vi "RedP--reader--V1.vi"() -> ()   [LabVIEW 2018]
uses:
  MFLI frontend action.ctl
  mfli reader event.ctl
  RedPitaSettings.ctl
  NHMFL_Core/Libraries/Red Pitaya/RP Core/RP Transceiver/RP Transceiver.lvclass
  publisher action.ctl
panel:
  in  "stop  !":bool
  in  "start  !":bool
  in  "all":enum32{"all"}(tab)
  out "read Voltage (V)":cdb=3.4008953474285613e-07-2.099650132525618e-08i format="%#10_10f"
  in  "read status":bool
  out "read Voltage X (V)":dbl=3.4008953474285613e-07 format="%#11_11f"
  out "read Voltage Y (V)":dbl=-2.099650132525618e-08 format="%#11_11f"
  in  "delay-read (msec)":u32=200
  out "zi freq (Hz)":dbl=59582.54261216211 format="%-#.3f"
  in  "red pita ip  Address":string="146.201.232.88"
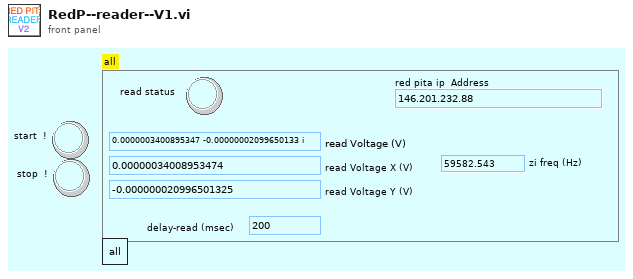
[diagram p1: front panel]
types:
  T1 = typedef "RedPitaSettings.ctl" = cluster{"time constant":dbl, "RP Transeiver":refnum<class "RP Transceiver.lvclass">, "samples per read":i32, "IP address":string}
  T2 = typedef "MFLI frontend action.ctl" = enum16{"read", "writeread", "open", "close", "write"}
  T3 = typedef "mfli reader event.ctl" = enum16{"start", "stop"}
  T4 = typedef "publisher action.ctl" = enum16{"set", "get", "init", "check"}
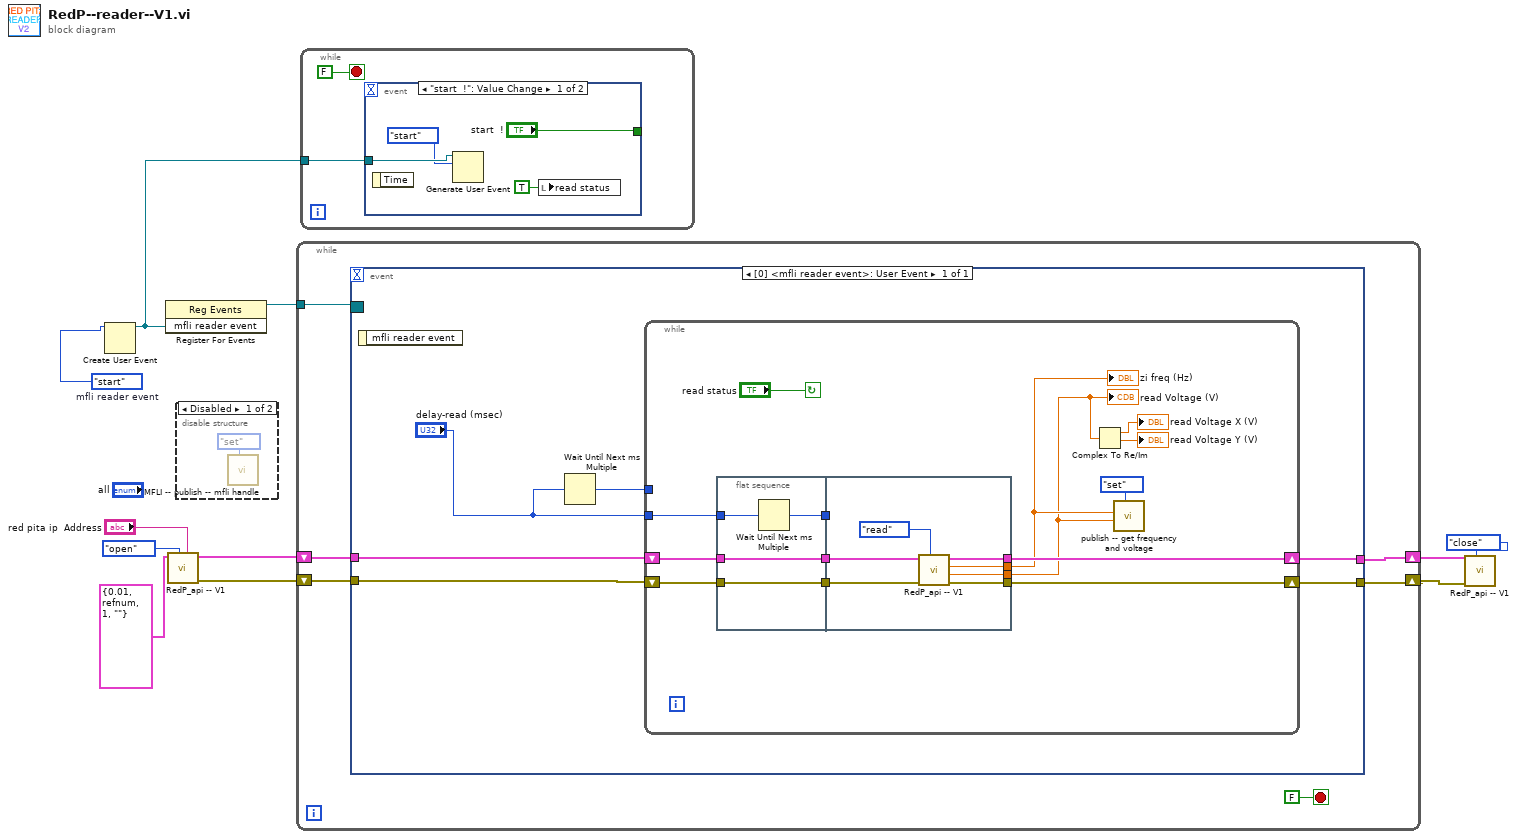
[diagram p0: block diagram]
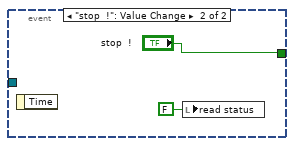
[diagram p3: hidden frame]
diagram:
  w8 = mfli_reader_event."start"  # mfli reader event
  n1 = Create User Event(user event datatype=w8) -> (user event=w7:refnum<user-event>)  [unwired: 1 in, 1 out]
  n2 = register-events(w7) -> (reference out=w9:refnum<event-registration>)  [unwired: 2 in, 1 out]
  n3 = call "RedP_api -- V1.vi"("red pita ip Address"="red pita ip  Address", "MFLI frontend action"=MFLI_frontend_action."open", "RedPitaSettings"=T1 {"time constant"=0.01, "RP Transeiver"=refnum, "samples per read"=1, "IP address"=""}) -> ("Error Out"=w2:errorcluster, "RedPitaSettings OUT"=w3:T1)  [unwired: 5 in, 2 out]
  n4 = disable-structure shown="Disabled" {
    frame Disabled {
      n5 = call "MFLI -- publish -- mfli handle.vi"("publisher action"=publisher_action."set") -> ()  [unwired: 10 in, 1 out]
    }
    frame Enabled {
    }
  }
  n6 = while {
    tunnel: w9 -> [w18]
    shift-right: [w16] -> w4
    shift-left: w3 -> [w15]
    shift-right: [w17] -> w5
    shift-left: w2 -> [w14]
    stop <- FALSE stop-if-true
    n7 = event shown="[0] <mfli reader event>: User Event" {
      selector: w18 -> [_]
      dyn-events: _ -> [_]
      timeout: _ -> [_]
      tunnel: w15 -> [w22]
      tunnel: w14 -> [w21]
      tunnel: [w24] -> w17
      tunnel: [w23] -> w16
      event User Event {
        n8 = event-data() -> ()  [unwired: 1 in, 1 out]
        n9 = Wait Until Next ms Multiple(millisecond multiple="delay-read (msec)") -> (millisecond timer value=w19:u32)
        n10 = while {
          shift-right: [w37] -> w24
          shift-left: w21 -> [w38]
          shift-right: [w35] -> w23
          shift-left: w22 -> [w36]
          tunnel: "delay-read (msec)" -> [w25]
          tunnel: w19 -> [_]
          stop <- "read status" continue-if-true
          n11 = flat-sequence {
            tunnel: [w42] -> w33
            tunnel: w25 -> [w41]
            tunnel: [w40] -> w32
            tunnel: w38 -> [w40]
            tunnel: w36 -> [w39]
            tunnel: [w39] -> w31
            tunnel: w33 -> [_]
            tunnel: [w47] -> w26
            tunnel: [w46] -> w27
            tunnel: w32 -> [w49]
            tunnel: [w48] -> w37
            tunnel: w31 -> [w43]
            tunnel: [w44] -> w35
            frame #0 {
              n12 = Wait Until Next ms Multiple(millisecond multiple=w41) -> (millisecond timer value=w42:u32)
            }
            frame #1 {
              n13 = call "RedP_api -- V1.vi"("MFLI frontend action"=MFLI_frontend_action."read", "Error In"=w49, "RedPitaSettings"=w43) -> ("Error Out"=w48:errorcluster, "z out (V)"=w47:cdb, "Freq out (Hz)"=w46:dbl, "RedPitaSettings OUT"=w44:T1)  [unwired: 5 in]
            }
          }
          n14 = Complex To Re/Im(x + iy=w26) -> (x=→"read Voltage X (V)":dbl, y=→"read Voltage Y (V)":dbl)
          n15 = call "publish -- get frequency and voltage.vi"("publisher action"=publisher_action."set", "Voltage IN (V)"=w26, "freq IN (Hz)"=w27) -> ()  [unwired: 6 in, 3 out]
          "read Voltage (V)" <- w26
          "zi freq (Hz)" <- w27
        }
      }
    }
  }
  n16 = while {
    tunnel: w7 -> [w51]
    stop <- FALSE stop-if-true
    n17 = event shown="[0] \"start  !\": Value Change" {
      selector: _ -> [_ _]
      dyn-events: _ -> [_ _]
      timeout: _ -> [_ _]
      tunnel: ["start  !" "stop  !"] -> _
      tunnel: w51 -> [w53 _]
      event "start  !": Value Change {
        n18 = event-data() -> ()  [unwired: 1 in, 1 out]
        n19 = Generate User Event(user event=w53, event data cluster=mfli_reader_event."start" ("event data")) -> ()  [unwired: 2 in, 2 out]
        n20 = local write "read status"(TRUE ("read status")) -> ()
      }
      event "stop  !": Value Change {
        n21 = event-data() -> ()  [unwired: 1 in, 1 out]
        n22 = local write "read status"(FALSE ("read status")) -> ()
      }
    }
  }
  n23 = call "RedP_api -- V1.vi"("MFLI frontend action"=MFLI_frontend_action."close", "Error In"=w5, "RedPitaSettings"=w4) -> ()  [unwired: 5 in, 4 out]
